vi "set_configuration_name.vi"(8 "error in (no error)":errorcluster, 10 "configuration":string, 11 "GenericPlugin.lvclass in":refnum<class "GenericComponent.lvclass">) -> (0 "error out":errorcluster, 3 "GenericPlugin.lvclass out":refnum<class "GenericComponent.lvclass">)   [LabVIEW 2010, in "GenericComponent.lvclass"]
uses:
  GenericComponent.lvclass
  GenericComponent.lvclass/GenericComponent.ctl
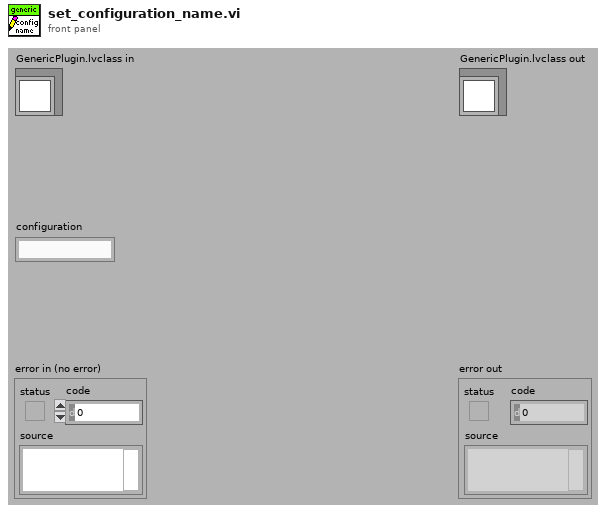
[diagram p1: front panel]
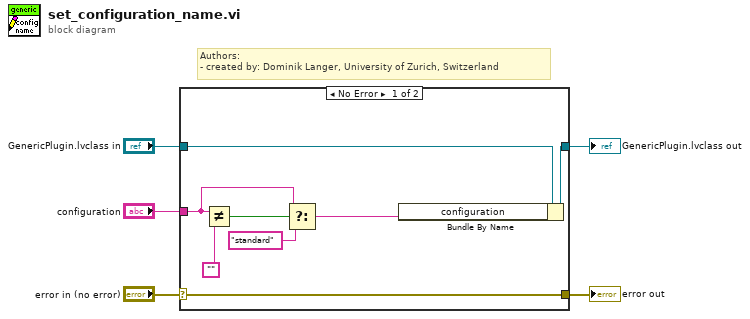
[diagram p0: block diagram]
diagram:
  # "Authors: \n- created by: Dominik Langer, University of Zurich, Switzerland"
  n1 = case shown="No Error" "error in (no error)" {
    selector: "error in (no error)" -> [w13 w14]
    tunnel: [w13 w14] -> w4
    tunnel: [w11 w15] -> w2
    tunnel: "GenericPlugin.lvclass in" -> [w12 w15]
    tunnel: "configuration" -> [w6 _]
    frame No Error {
      n2 = Not Equal?(x=w6, y="") -> (x != y?=w8:bool)
      n3 = Select(t=w6, s=w8, f="standard") -> (s? t:f=w7:string)
      n4 = Bundle By Name(cluster=w12, "configuration"=w7) -> (w11:refnum<class "GenericComponent.lvclass">)
    }
    frame Error {
    }
  }
  "error out" <- w4
  "GenericPlugin.lvclass out" <- w2
